vi "joystick control debugging.vi"() -> ()   [LabVIEW 2014]
uses:
  <vilib>/Utility/inputDevices.llb/joystickAcquire.vi
  <vilib>/Utility/inputDevices.llb/closeJoystick.vi
panel:
  out "device ID":refnum<k1>
  out "button info":T1
  out "device ID 2":refnum<k1>
  out "Value":T2(ring)
  out "JoystOffset":T3={"XOffset"=-99999, "YOffset"=-99999, "ZOffset"=-99999}
  out "RelJoyPos":T4
  in  "XMotorRef":refnum<k7>(container)
  in  "YMotorRef":refnum<k7>(container)
  in  "ZMotorRef":refnum<k7>(container)
  out "joystick info":T5(array[cluster])
  out "InstrumentMode":T2(ring)=enum."Shutdown"
  in  "InterfaceSelector":T6(tab)
  in  "GoToTopDisp":bool
  in  "GoToBottDisp":bool
  in  "GoToExpLoc":bool
  in  "SaveTopDisp":bool
  in  "SaveBottDisp":bool
  in  "SaveExpLoc":bool
  out "Top Dispenser":T7={"X Pos (mm)"=0.5532008, "Y Pos (mm)"=0.030929338, "Z Pos (mm)"=0.77973413} {"Y Pos (mm)" format="%.3f"; "Z Pos (mm)" format="%.3f"; "X Pos (mm)" format="%.3f"}
  out "Bottom Dispenser":T7={"X Pos (mm)"=0.600309, "Y Pos (mm)"=-1.1540928, "Z Pos (mm)"=0.7938141} {"Y Pos (mm)" format="%.3f"; "Z Pos (mm)" format="%.3f"; "X Pos (mm)" format="%.3f"}
  out "Experiment Region":T7={"X Pos (mm)"=1.4278219, "Y Pos (mm)"=-0.74810517, "Z Pos (mm)"=0.7938141} {"Y Pos (mm)" format="%.3f"; "Z Pos (mm)" format="%.3f"; "X Pos (mm)" format="%.3f"}
  in  "PreviewPanel":T8(tab)
  in  "Z Motor Settings":T9={"Joyst Min Signal"=10.0, "Joyst Max Signal"=30000.0, "Vmax (mm/s)"=0.005, "Acc (mm/s/s)"=0.2, "+ JoystDirection"=2, "- JoystDirection"=1} {"Acc (mm/s/s)" format="%#.3f"; "Vmax (mm/s)" format="%#.3f"}
  in  "Y Motor Settings":T9={"Joyst Min Signal"=10.0, "Joyst Max Signal"=20000.0, "Vmax (mm/s)"=0.03, "Acc (mm/s/s)"=0.5, "+ JoystDirection"=1, "- JoystDirection"=2} {"Acc (mm/s/s)" format="%#.3f"; "Vmax (mm/s)" format="%#.3f"}
  in  "X Motor Settings":T9={"Joyst Min Signal"=10.0, "Joyst Max Signal"=20000.0, "Vmax (mm/s)"=0.03, "Acc (mm/s/s)"=0.5, "+ JoystDirection"=2, "- JoystDirection"=1} {"Acc (mm/s/s)" format="%#.3f"; "Vmax (mm/s)" format="%#.3f"}
  in  "Motor Cruise Param":T10={"X Acc (mm/s^2)"=0.3, "X Vmax (mm/s)"=0.3, "Y Acc (mm/s^2)"=0.3, "Y Vmax (mm/s)"=0.3, "Z Acc (mm/s^2)"=0.1, "Z Vmax (mm/s)"=0.1}
  in  "Motor Limits":T11={"XMin"=-0.8, "XMax"=3.0, "YMin"=-2.0, "YMax"=2.0, "ZMin"=0.0, "ZMax"=2.0}
  in  "Steerable Mirror Calibration":T12={"Hor. Scaling (nm/V)"=760.0, "Vert. Scaling (nm/V)"=760.0, "Hor. Mirr. Offset (V)"=0.0, "Vert. Mirr. Offset (V)"=0.0}
  in  "Steerable \nTrap\n(F12)":bool
  in  "Fixed\nTrap\n(F11)":bool
  in  "Align Traps Vertically":bool
  in  "MaxHorizontalTrapSeparation":bool
  out "X Motor State":T13={"Direction"=0, "Vel (mm/s)"=0.0, "IsActive?"=FALSE, "Pos (mm)"=-0.2957381} {"Pos (mm)" format="%#.3f"; "Vel (mm/s)" format="%#.4f"}
  out "Y Motor State":T13={"Direction"=0, "Vel (mm/s)"=0.0, "IsActive?"=FALSE, "Pos (mm)"=0.016441232} {"Pos (mm)" format="%#.3f"; "Vel (mm/s)" format="%#.4f"}
  out "Z Motor State":T13={"Direction"=0, "Vel (mm/s)"=0.0, "IsActive?"=FALSE, "Pos (mm)"=-0.26253498} {"Pos (mm)" format="%#.3f"; "Vel (mm/s)" format="%#.4f"}
  out "Move Z":bool
  out "Move XY":bool
  in  "MotorLoopDelay":u32=100
  in  "PMVertSlider(V)":dbl(slide)=0.005145263671875 scale=0.0..10.0 scale format="%#_3f"
  in  "PMHorizSlider(V)":dbl(slide)=0.0045623779296875 scale=2.0..10.0
  out "Force TrapA":cluster{"x":dbl[], "y":dbl[]}[](graph)
  out "Noise-Ext":cluster{"x":dbl[], "y":dbl[]}[](graph)
  out "Force TrapB":cluster{"x":dbl[], "y":dbl[]}[](graph)
  out "IsOffsetModeActive?":bool caption="stop"
  # "Chamber Locations"
  # "Need a Button Here that would read the \nNormalized Offset and save it"
  # "Off"
  # "On"
  # "Off"
  # "On"
  # "Thorlabs Motor Status"
  # "Passive Mode"
  # "when I switch tabs from the passive mode to basic mode, the recording doesn't stop"
  # "The sliders don't do anything in passive mode, fix it"
  # "Whenever I click on Ackquire Offset, it goes back to the basic operation, then I have to ckick again"
  # "Trap Motion Control"
  # "Steerable Mirror Info"
  # "Zero-Force Offset Mode"
  # "High Frequency Data Acquisition"
  # "Adjust the length of acquisition time"
  # "Force-Extension Mode"
  # "Y"
  # "+"
  # "X"
  # "-"
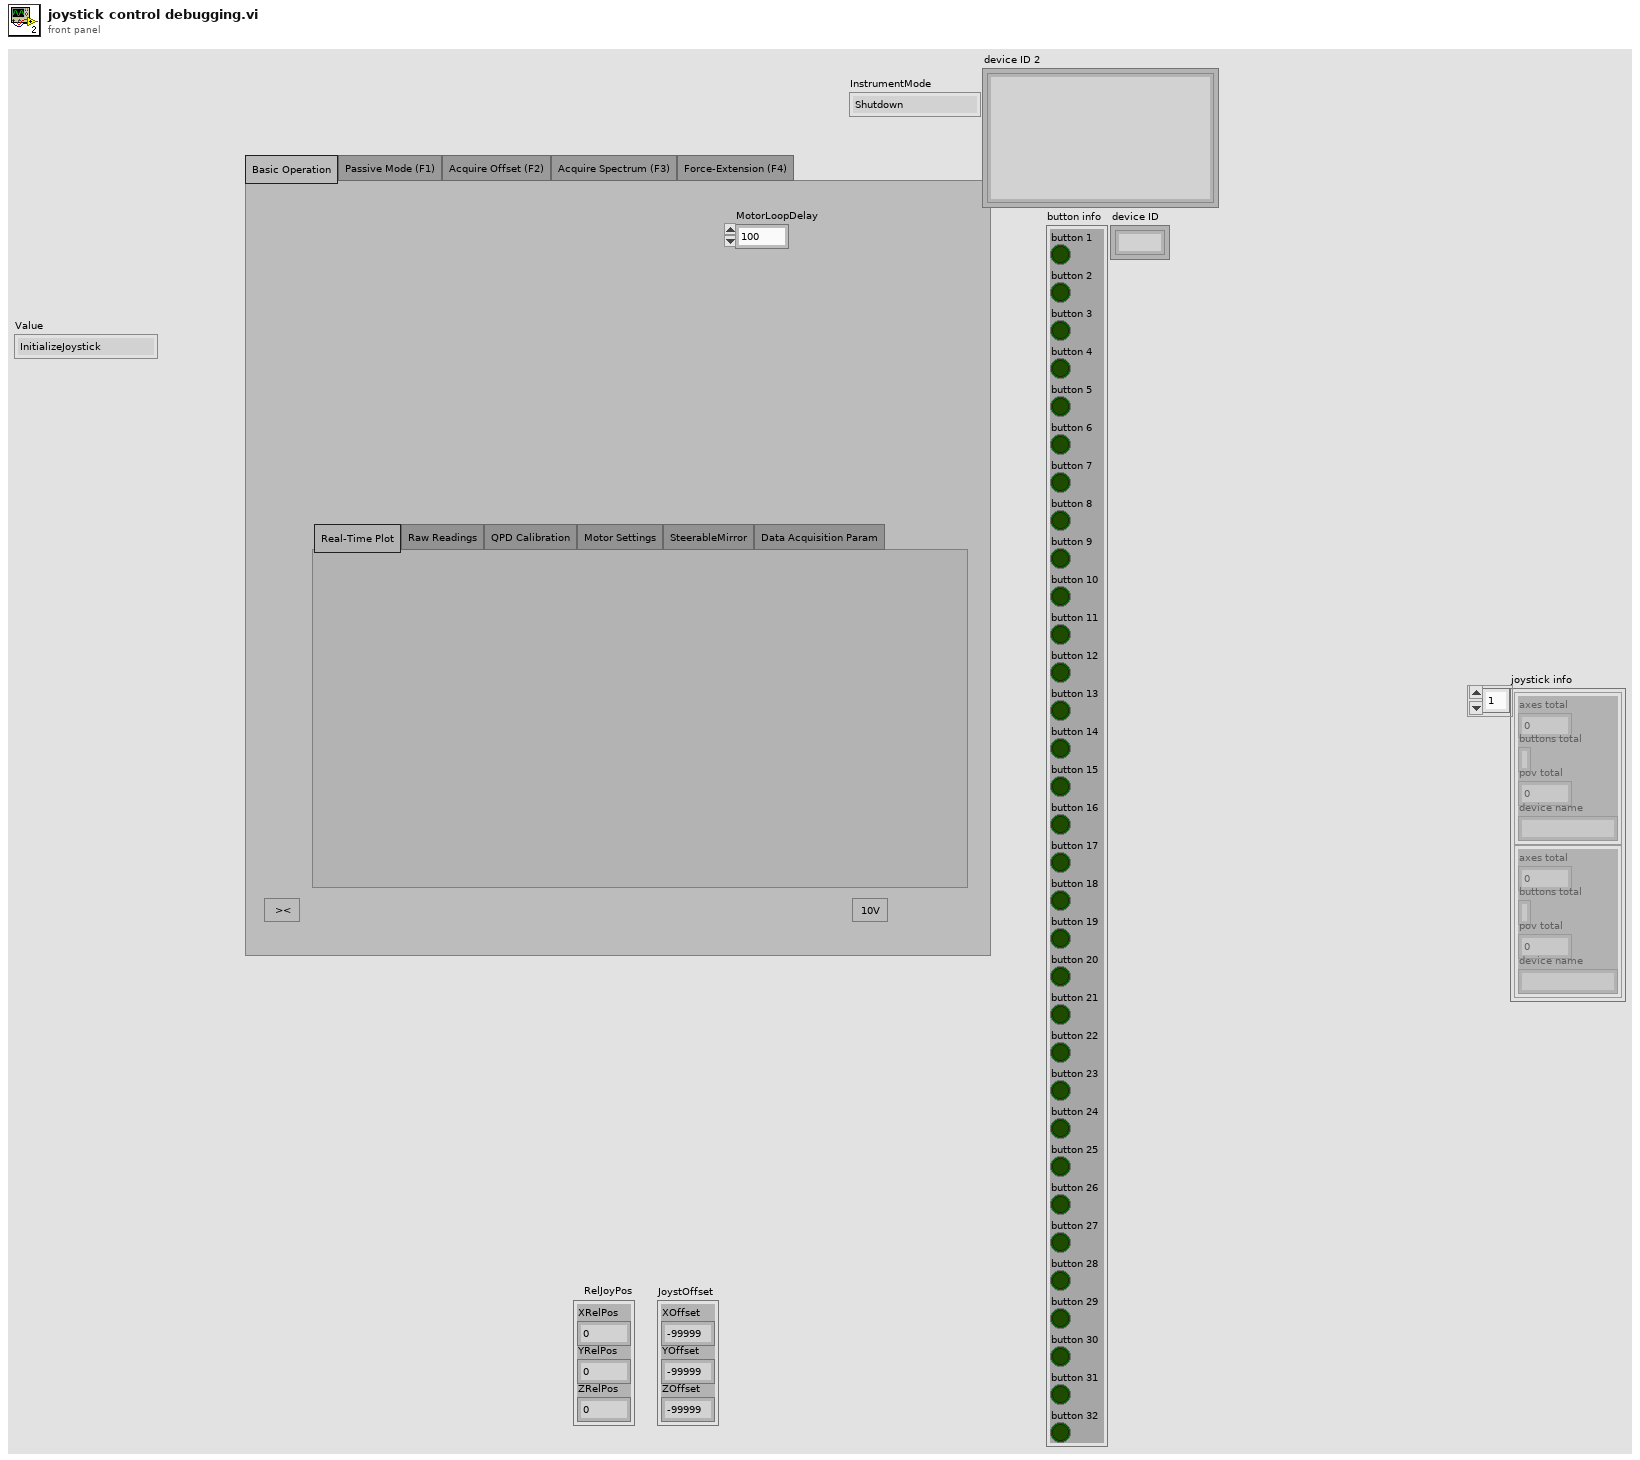
[diagram p1: front panel]
types:
  T1 = cluster{"button 1":bool, "button 2":bool, "button 3":bool, "button 4":bool, "button 5":bool, "button 6":bool, "button 7":bool, "button 8":bool, "button 9":bool, "button 10":bool, "button 11":bool, "button 12":bool, "button 13":bool, "button 14":bool, "button 15":bool, "button 16":bool, "button 17":bool, "button 18":bool, "button 19":bool, "button 20":bool, "button 21":bool, "button 22":bool, "button 23":bool, "button 24":bool, "button 25":bool, "button 26":bool, "button 27":bool, "button 28":bool, "button 29":bool, "button 30":bool, "button 31":bool, "button 32":bool}
  T2 = enum16{"InitializeJoystick", "InitializeMotors", "BasicMode", "PassiveMode", "AcquireOffsetMode", "AcquireSpectrumMode", "Force-ExtensionMode", "Shutdown"}
  T3 = cluster{"XOffset":i32, "YOffset":i32, "ZOffset":i32}
  T4 = cluster{"XRelPos":i32, "YRelPos":i32, "ZRelPos":i32}
  T5 = cluster{"axes total":u32, "buttons total":u32, "pov total":u32, "device name":string}[]
  T6 = enum32{"Basic Operation", "Passive Mode (F1)", "Acquire Offset (F2)", "Acquire Spectrum (F3)", "Force-Extension (F4)"}
  T7 = cluster{"X Pos (mm)":sgl, "Y Pos (mm)":sgl, "Z Pos (mm)":sgl}
  T8 = enum32{"Real-Time Plot", "Raw Readings", "QPD Calibration", "Motor Settings", "SteerableMirror", "Data Acquisition Param"}
  T9 = cluster{"Joyst Min Signal":dbl, "Joyst Max Signal":dbl, "Vmax (mm/s)":sgl, "Acc (mm/s/s)":sgl, "+ JoystDirection":i32, "- JoystDirection":i32}
  T10 = cluster{"X Acc (mm/s^2)":sgl, "X Vmax (mm/s)":sgl, "Y Acc (mm/s^2)":sgl, "Y Vmax (mm/s)":sgl, "Z Acc (mm/s^2)":sgl, "Z Vmax (mm/s)":sgl}
  T11 = cluster{"XMin":sgl, "XMax":sgl, "YMin":sgl, "YMax":sgl, "ZMin":sgl, "ZMax":sgl}
  T12 = cluster{"Hor. Scaling (nm/V)":dbl, "Vert. Scaling (nm/V)":dbl, "Hor. Mirr. Offset (V)":dbl, "Vert. Mirr. Offset (V)":dbl}
  T13 = cluster{"Direction":i32, "Vel (mm/s)":sgl, "IsActive?":bool, "Pos (mm)":sgl}
  T14 = cluster{"Motor Reference":refnum<k7>, "Motor Reference":refnum<k7>, "Motor Reference":refnum<k7>}
  T15 = cluster{"X axis":i32, "Y axis":i32, "Z axis":i32, "X axis rotation":i32, "Y axis rotation":i32, "Z axis rotation":i32, "U axis":i32, "V axis":i32}
  T16 = cluster{"XMotorRef":refnum<k7>, "YMotorRef":refnum<k7>, "ZMotorRef":refnum<k7>}
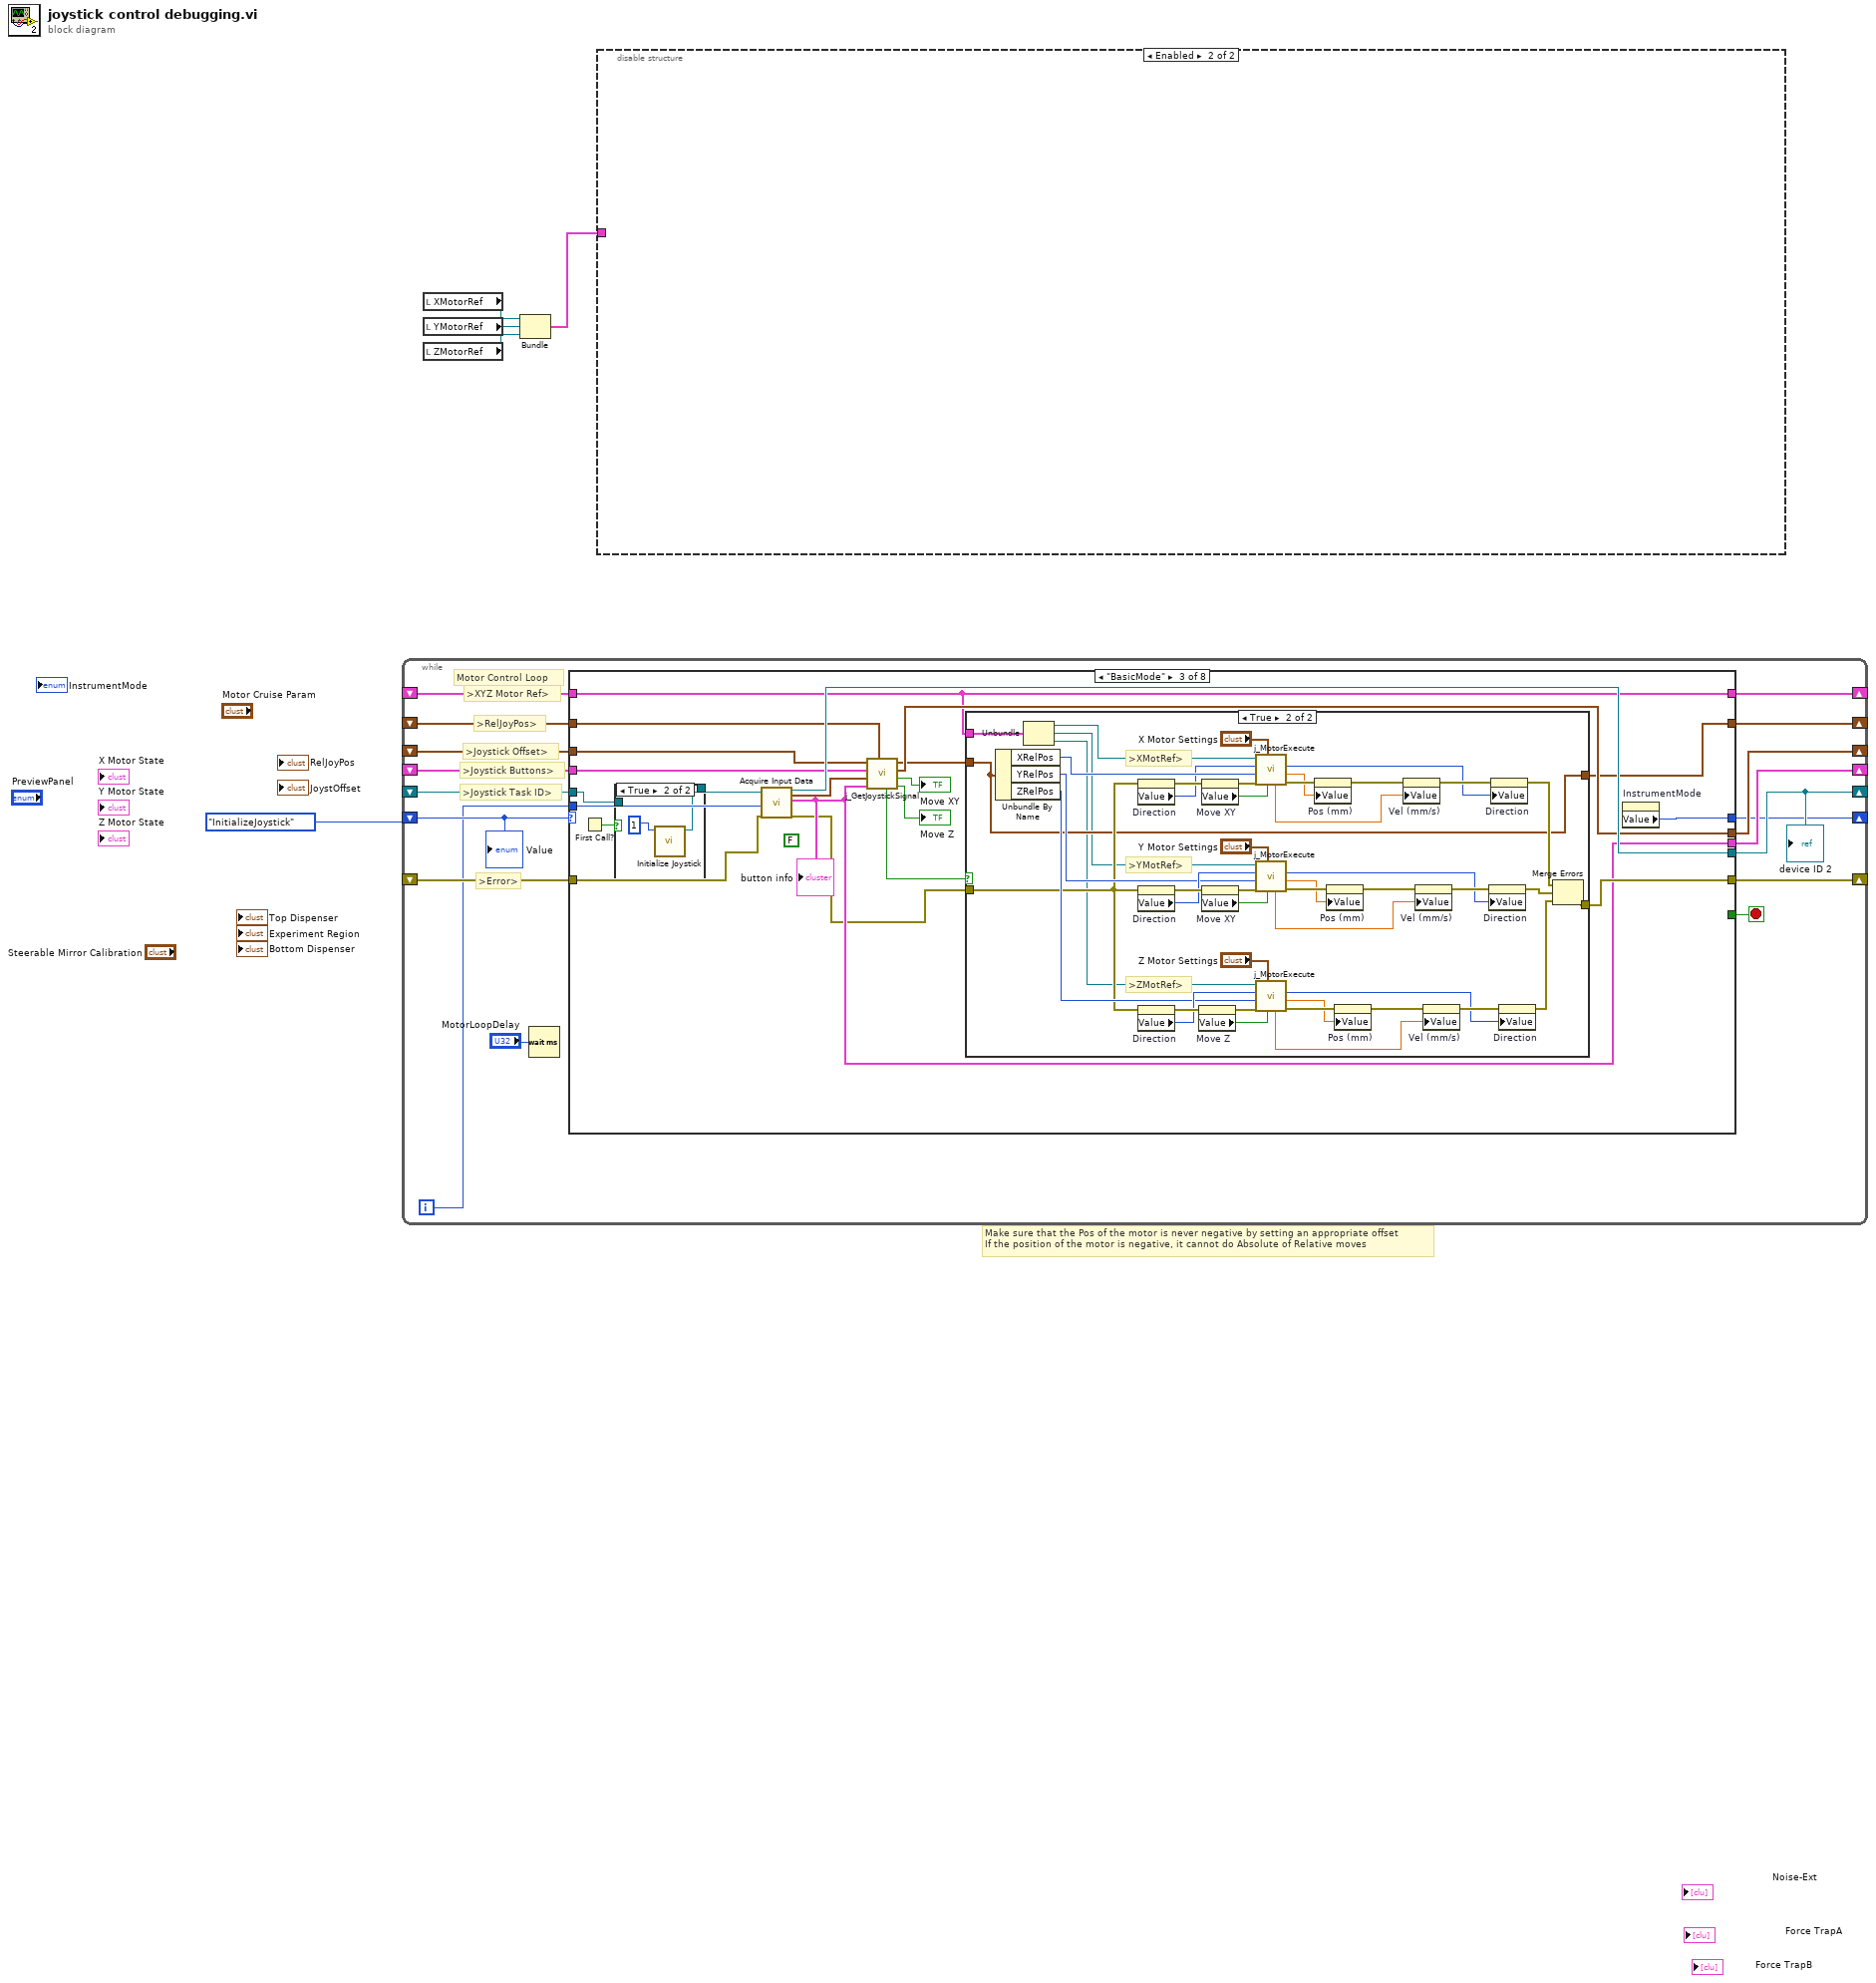
[diagram p0: block diagram]
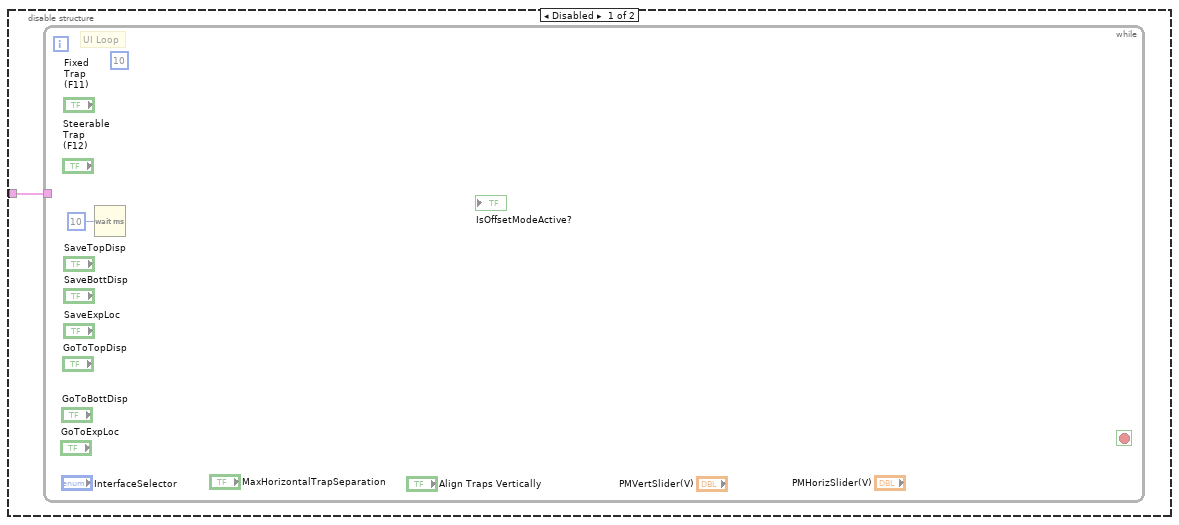
[diagram p2: hidden frame]
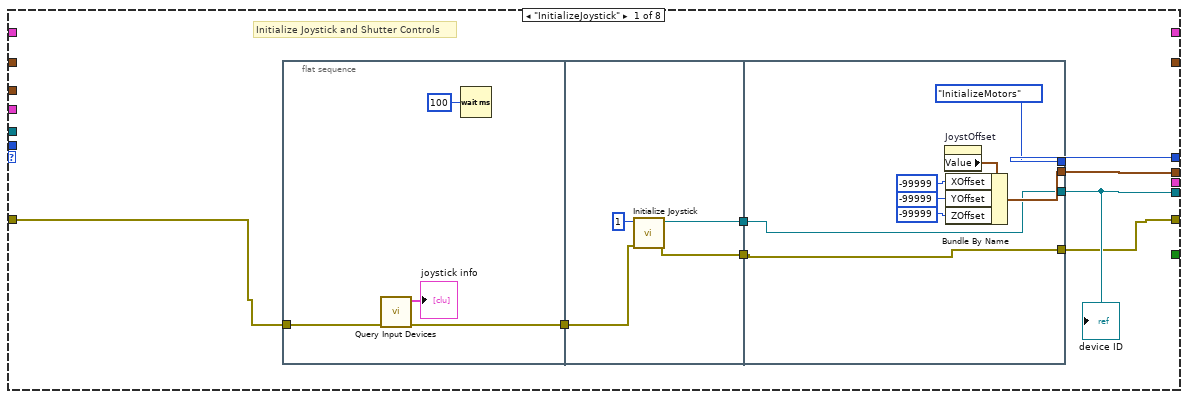
[diagram p3: hidden frame]
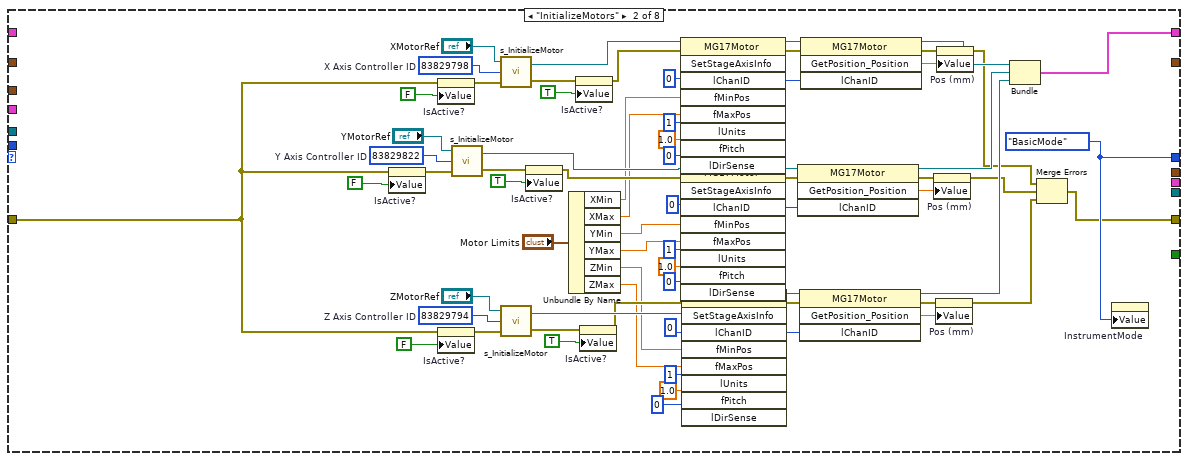
[diagram p4: hidden frame]
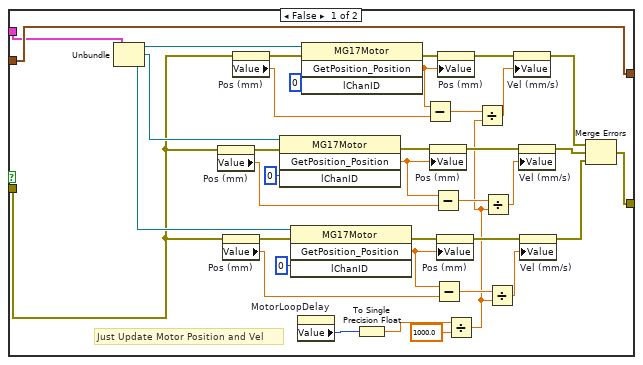
[diagram p6: hidden frame]
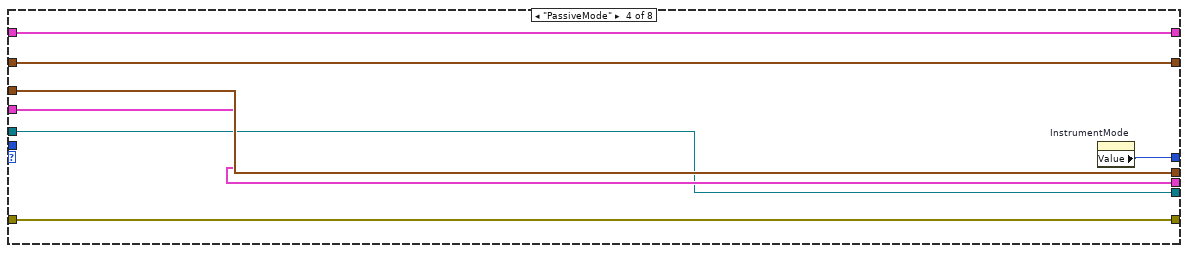
[diagram p7: hidden frame]
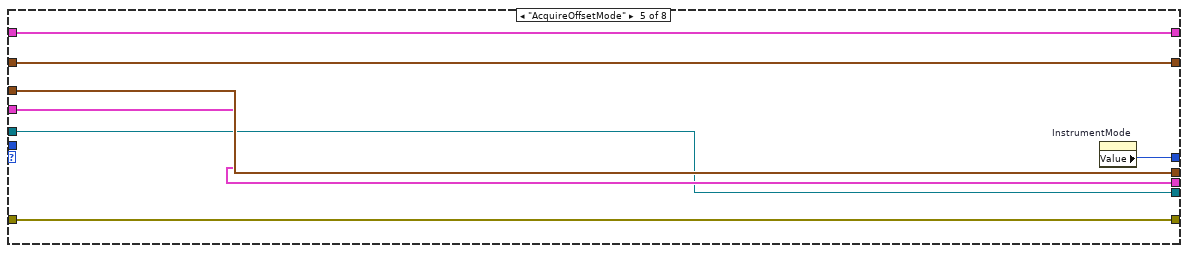
[diagram p8: hidden frame]
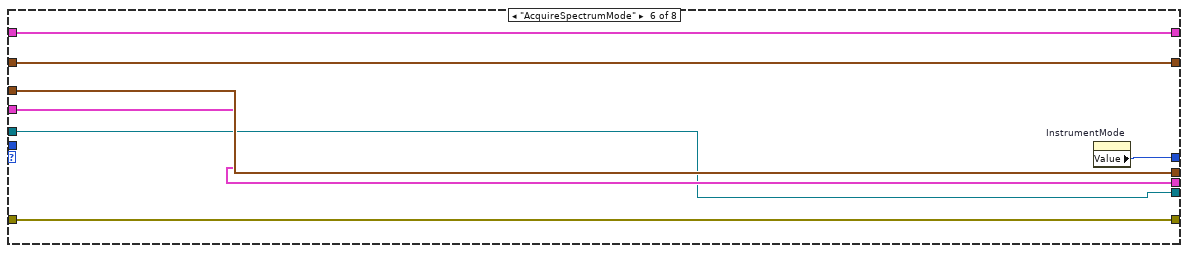
[diagram p9: hidden frame]
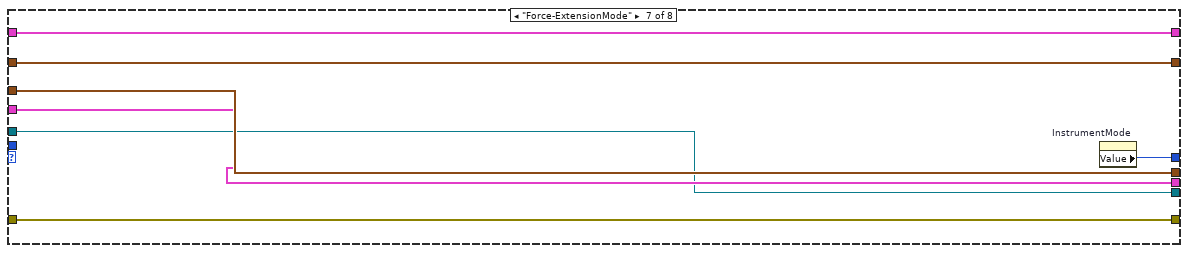
[diagram p10: hidden frame]
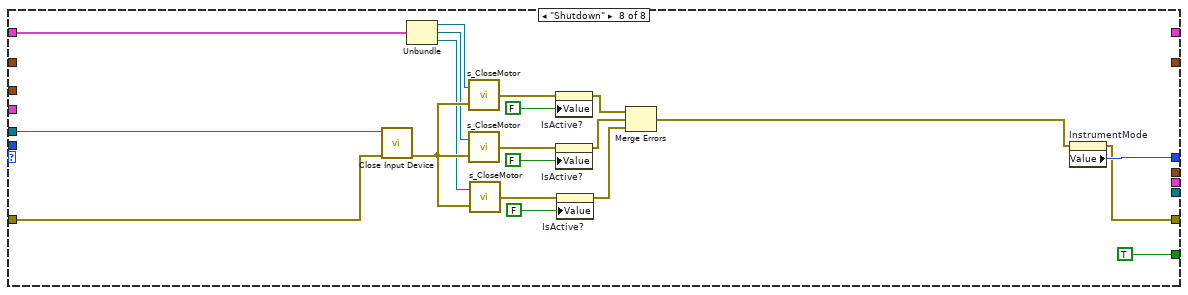
[diagram p11: hidden frame]
diagram:
  # "Make sure that the Pos of the motor is never negative by setting an appropriate offset\nIf the position of the motor is negative, it cannot do Absolute of Relative moves"
  n1 = while {
    shift-right: [w8] -> _
    shift-left: T2."InitializeJoystick" -> [w7]
    shift-right: [w22] -> _
    shift-left: _ -> [w15]
    shift-right: [w19] -> _
    shift-left: _ -> [w21]
    shift-right: [w20] -> _
    shift-left: _ -> [w18]
    shift-right: [w17] -> _
    shift-left: _ -> [w16]
    shift-right: [w14] -> _
    shift-left: _ -> [w11]
    shift-right: [w12] -> _
    shift-left: _ -> [w13]
    i -> [w6]
    stop <- w9 stop-if-true
    # "Motor Control Loop"
    # ">Joystick Offset>"
    # ">RelJoyPos>"
    # ">XYZ Motor Ref>"
    # ">Error>"
    # ">Joystick Task ID>"
    # ">Joystick Buttons>"
    n2 = Wait (ms)(milliseconds to wait="MotorLoopDelay") -> ()  [unwired: 1 out]
    n3 = case shown="\"BasicMode\"" w7 {
      tunnel: [w30 _ w133 w225 w232 w239 w246 _] -> w22
      tunnel: [w28 w48 w122 w229 w236 w243 w250 w269] -> w8
      tunnel: w21 -> [w27 w96 w135 w228 w235 w242 w249 w254]
      tunnel: [w29 _ w134 w223 w230 w237 w244 _] -> w20
      tunnel: [w26 w47 w126 w228 w235 w242 w249 w251] -> w19
      tunnel: w18 -> [_ _ w115 w223 w230 w237 w244 w253]
      tunnel: [_ _ w121 w224 w231 w238 w245 _] -> w17
      tunnel: w16 -> [_ _ w120 w224 w231 w238 w245 _]
      tunnel: w15 -> [_ _ w131 w225 w232 w239 w246 _]
      tunnel: [_ _ _ _ _ _ _ TRUE ("status")] -> w9
      tunnel: [_ w95 w125 w227 w234 w241 w248 _] -> w14
      tunnel: w11 -> [_ _ w125 w227 w234 w241 w248 w255]
      tunnel: [_ _ w123 w226 w233 w240 w247 _] -> w12
      tunnel: w13 -> [_ _ w132 w226 w233 w240 w247 _]
      tunnel: w6 -> [_ _ w118 _ _ _ _ _]
      frame "InitializeJoystick" {
        # "Initialize Joystick and Shutter Controls"
        n4 = flat-sequence {
          tunnel: w27 -> [w32]
          tunnel: [w31] -> w25
          tunnel: w25 -> [w37]
          tunnel: [w36] -> w24
          tunnel: [w35] -> w23
          tunnel: [w43] -> w30
          tunnel: [w39] -> w29
          tunnel: [T2."InitializeMotors"] -> w28
          tunnel: w24 -> [w40]
          tunnel: [w40] -> w26
          tunnel: w23 -> [w39]
          frame #0 {
            n5 = call <vilib>:"Query Input Devices.vi"("error in (no error)"=w32) -> ("error out"=w31:errorcluster, "joystick info"=→"joystick info":T5)  [unwired: 7 in, 2 out]
            n6 = Wait (ms)(milliseconds to wait=u32 100) -> ()  [unwired: 1 out]
          }
          frame #1 {
            n7 = call <vilib>:"Initialize Joystick.vi"("error in (no error)"=w37, "device index"=1) -> ("error out"=w36:errorcluster, "device ID"=w35:refnum<k1>)  [unwired: 8 in]
          }
          frame #2 {
            n8 = property on="JoystOffset" class="Clust (strict)"() -> ("Value"=w42:T3)  [unwired: 2 in, 2 out]
            n9 = Bundle By Name(cluster=w42, "XOffset"=-99999, "YOffset"=-99999, "ZOffset"=-99999) -> (w43:T3)
          }
        }
        "device ID" <- w29
      }
      frame "InitializeMotors" {
        w48 = T2."BasicMode"
        w100 = 83829794  # Z Axis Controller ID
        w106 = 83829822  # Y Axis Controller ID
        w112 = 83829798  # X Axis Controller ID
        n10 = property on="IsActive?" class="Bool (strict)"(error in=w96, "Value"=FALSE ("IsYMotorActive?")) -> (error out=w107:errorcluster)  [unwired: 1 in, 1 out]
        n11 = property on="IsActive?" class="Bool (strict)"(error in=w96, "Value"=FALSE ("IsYMotorActive?")) -> (error out=w113:errorcluster)  [unwired: 1 in, 1 out]
        n12 = property on="IsActive?" class="Bool (strict)"(error in=w96, "Value"=FALSE ("IsYMotorActive?")) -> (error out=w101:errorcluster)  [unwired: 1 in, 1 out]
        n13 = call "s_InitializeMotor.vi"("Error In"=w107, "Servo Controller  ID"=w106, "Motor Reference In"="YMotorRef") -> ("Error Out"=w108:errorcluster, "Motor Reference"=w90:refnum<k7>)
        n14 = call "s_InitializeMotor.vi"("Error In"=w113, "Servo Controller  ID"=w112, "Motor Reference In"="XMotorRef") -> ("Error Out"=w114:errorcluster, "Motor Reference"=w94:refnum<k7>)
        n15 = call "s_InitializeMotor.vi"("Error In"=w101, "Servo Controller  ID"=w100, "Motor Reference In"="ZMotorRef") -> ("Error Out"=w102:errorcluster, "Motor Reference"=w87:refnum<k7>)
        n16 = property on="IsActive?" class="Bool (strict)"(error in=w108, "Value"=TRUE ("IsYMotorActive?")) -> (error out=w89:errorcluster)  [unwired: 1 in, 1 out]
        n17 = Unbundle By Name("Motor Limits") -> ("XMin"=w54:sgl, "XMax"=w53:sgl, "YMin"=w52:sgl, "YMax"=w51:sgl, "ZMin"=w50:sgl, "ZMax"=w49:sgl)
        n18 = property on="IsActive?" class="Bool (strict)"(error in=w114, "Value"=TRUE ("IsYMotorActive?")) -> (error out=w92:errorcluster)  [unwired: 1 in, 1 out]
        n19 = property on="IsActive?" class="Bool (strict)"(error in=w102, "Value"=TRUE ("IsYMotorActive?")) -> (error out=w86:errorcluster)  [unwired: 1 in, 1 out]
        n20 = invoke class="MG17Motor" method="SetStageAxisInfo"(reference=w94, error in=w92, "lChanID"=0, "fMinPos"=w54, "fMaxPos"=w53, "lUnits"=1, "fPitch"=sgl 1.0, "lDirSense"=0) -> (reference out=w85:refnum<k7>, error out=w84:errorcluster, "lChanID"=w83:i32)  [unwired: 1 in, 6 out]
        n21 = invoke class="MG17Motor" method="SetStageAxisInfo"(reference=w90, error in=w89, "lChanID"=0, "fMinPos"=w52, "fMaxPos"=w51, "lUnits"=1, "fPitch"=sgl 1.0, "lDirSense"=0) -> (reference out=w77:refnum<k7>, error out=w76:errorcluster, "lChanID"=w75:i32)  [unwired: 1 in, 6 out]
        n22 = invoke class="MG17Motor" method="SetStageAxisInfo"(reference=w87, error in=w86, "lChanID"=0, "fMinPos"=w50, "fMaxPos"=w49, "lUnits"=1, "fPitch"=sgl 1.0, "lDirSense"=0) -> (reference out=w72:refnum<k7>, error out=w71:errorcluster, "lChanID"=w70:i32)  [unwired: 1 in, 6 out]
        n23 = invoke class="MG17Motor" method="GetPosition_Position"(reference=w77, error in=w76, "lChanID"=w75) -> (reference out=w69:refnum<k7>, error out=w79:errorcluster, "GetPosition_Position"=w78:sgl)  [unwired: 1 in, 1 out]
        n24 = invoke class="MG17Motor" method="GetPosition_Position"(reference=w72, error in=w71, "lChanID"=w70) -> (reference out=w68:refnum<k7>, error out=w74:errorcluster, "GetPosition_Position"=w73:sgl)  [unwired: 1 in, 1 out]
        n25 = invoke class="MG17Motor" method="GetPosition_Position"(reference=w85, error in=w84, "lChanID"=w83) -> (reference out=w82:refnum<k7>, error out=w81:errorcluster, "GetPosition_Position"=w80:sgl)  [unwired: 1 in, 1 out]
        n26 = property on="Pos (mm)" class="DigNum (strict)"(error in=w79, "Value"=w78) -> (error out=w67:errorcluster)  [unwired: 1 in, 1 out]
        n27 = property on="Pos (mm)" class="DigNum (strict)"(error in=w74, "Value"=w73) -> (error out=w65:errorcluster)  [unwired: 1 in, 1 out]
        n28 = property on="Pos (mm)" class="DigNum (strict)"(error in=w81, "Value"=w80) -> (error out=w66:errorcluster)  [unwired: 1 in, 1 out]
        n29 = Bundle("Motor Reference"=w82, "Motor Reference"=w69, "Motor Reference"=w68) -> (w95:T14)  [unwired: 1 in]
        n30 = Merge Errors(w66, w67, w65) -> (w47:errorcluster)
        n31 = property on="InstrumentMode" class="Enum (strict)"("Value"=w48) -> ()  [unwired: 2 in, 2 out]
      }
      frame "BasicMode" {
        (unwired) FALSE
        n32 = First Call?() -> (First Call?: T/F=w116:bool)
        n33 = case shown="True" w116 {
          tunnel: [w136 w137] -> w117
          tunnel: w115 -> [w136 _]
          frame False {
          }
          frame True {
            n34 = call <vilib>:"Initialize Joystick.vi"("device index"=1) -> ("device ID"=w137:refnum<k1>)  [unwired: 9 in, 1 out]
          }
        }
        n35 = call-poly <vilib>:"Acquire Input Data.vi"("device ID"=w117, "Numeric"=w118, "error in (no error)"=w135) -> ("device ID 2"=w134:refnum<k1>, "axis info"=w130:T15, "button info"=w121:T1, "error out"=w119:errorcluster)  [unwired: 12 in, 1 out]
        "button info" <- w121
        n36 = call "j_GetJoystickSignal.vi"("RelJoyPos In"=w132, "NewJoystButtInfo"=w121, "NewJoystAxisInfo"=w130, "OldJoystButtInfo"=w120, "OldJoystickOffset"=w131) -> ("MoveZ"=→"Move Z":bool, "MoveXY"=→"Move XY":bool, "Joystick Offset"=w133:T3, "RelJoyPos"=w127:T4, "TalkToMotors?"=w124:bool)
        n37 = case shown="True" w124 {
          tunnel: w127 -> [w176 w180]
          tunnel: [w165 w197] -> w126
          tunnel: w125 -> [w175 w183]
          tunnel: w119 -> [w149 w182]
          tunnel: [w176 w180] -> w123
          frame False {
            # "Just Update Motor Position and Vel"
            n38 = Unbundle(w175) -> ("Motor Reference"=w174:refnum<k7>, "Motor Reference"=w167:refnum<k7>, "Motor Reference"=w166:refnum<k7>)
            n39 = property on="Pos (mm)" class="DigNum (strict)"(error in=w149) -> (error out=w157:errorcluster, "Value"=w154:sgl)  [unwired: 1 in, 1 out]
            n40 = property on="Pos (mm)" class="DigNum (strict)"(error in=w149) -> (error out=w150:errorcluster, "Value"=w147:sgl)  [unwired: 1 in, 1 out]
            n41 = property on="Pos (mm)" class="DigNum (strict)"(error in=w149) -> (error out=w158:errorcluster, "Value"=w163:sgl)  [unwired: 1 in, 1 out]
            n42 = invoke class="MG17Motor" method="GetPosition_Position"(reference=w167, error in=w157, "lChanID"=0) -> (error out=w170:errorcluster, "GetPosition_Position"=w155:sgl)  [unwired: 1 in, 2 out]
            n43 = invoke class="MG17Motor" method="GetPosition_Position"(reference=w166, error in=w150, "lChanID"=0) -> (error out=w168:errorcluster, "GetPosition_Position"=w146:sgl)  [unwired: 1 in, 2 out]
            n44 = property on="MotorLoopDelay" class="DigNum (strict)"() -> ("Value"=w142:u32)  [unwired: 2 in, 2 out]
            n45 = invoke class="MG17Motor" method="GetPosition_Position"(reference=w174, error in=w158, "lChanID"=0) -> (error out=w172:errorcluster, "GetPosition_Position"=w164:sgl)  [unwired: 1 in, 2 out]
            n46 = To Single Precision Float(number=w142) -> (single precision float=w141:sgl)
            n47 = Subtract(x=w164, y=w163) -> (x-y=w162:sgl)
            n48 = property on="Pos (mm)" class="DigNum (strict)"(error in=w170, "Value"=w155) -> (error out=w153:errorcluster)  [unwired: 1 in, 1 out]
            n49 = Subtract(x=w155, y=w154) -> (x-y=w156:sgl)
            n50 = Subtract(x=w146, y=w147) -> (x-y=w148:sgl)
            n51 = property on="Pos (mm)" class="DigNum (strict)"(error in=w168, "Value"=w146) -> (error out=w145:errorcluster)  [unwired: 1 in, 1 out]
            n52 = property on="Pos (mm)" class="DigNum (strict)"(error in=w172, "Value"=w164) -> (error out=w160:errorcluster)  [unwired: 1 in, 1 out]
            n53 = Divide(x=w141, y=sgl 1000.0) -> (x/y=w139:sgl)
            n54 = Divide(x=w162, y=w139) -> (x/y=w161:sgl)
            n55 = Divide(x=w156, y=w139) -> (x/y=w152:sgl)
            n56 = Divide(x=w148, y=w139) -> (x/y=w144:sgl)
            n57 = property on="Vel (mm/s)" class="DigNum (strict)"(error in=w160, "Value"=w161) -> (error out=w159:errorcluster)  [unwired: 1 in, 1 out]
            n58 = property on="Vel (mm/s)" class="DigNum (strict)"(error in=w153, "Value"=w152) -> (error out=w151:errorcluster)  [unwired: 1 in, 1 out]
            n59 = property on="Vel (mm/s)" class="DigNum (strict)"(error in=w145, "Value"=w144) -> (error out=w143:errorcluster)  [unwired: 1 in, 1 out]
            n60 = Merge Errors(w159, w151, w143) -> (w165:errorcluster)
          }
          frame True {
            # ">ZMotRef>"
            # ">YMotRef>"
            # ">XMotRef>"
            n61 = Unbundle By Name(w180) -> ("XRelPos"=w213:i32, "YRelPos"=w199:i32, "ZRelPos"=w184:i32)
            n62 = Unbundle(w183) -> ("Motor Reference"=w179:refnum<k7>, "Motor Reference"=w178:refnum<k7>, "Motor Reference"=w177:refnum<k7>)
            n63 = property on="Direction" class="DigNum (strict)"(error in=w182) -> (error out=w212:errorcluster, "Value"=w211:i32)  [unwired: 1 in, 1 out]
            n64 = property on="Direction" class="DigNum (strict)"(error in=w182) -> (error out=w202:errorcluster, "Value"=w201:i32)  [unwired: 1 in, 1 out]
            n65 = property on="Direction" class="DigNum (strict)"(error in=w182) -> (error out=w187:errorcluster, "Value"=w186:i32)  [unwired: 1 in, 1 out]
            n66 = property on="Move Z" class="Bool (strict)"(error in=w187) -> (error out=w195:errorcluster, "Value"=w194:bool)  [unwired: 1 in, 1 out]
            n67 = property on="Move XY" class="Bool (strict)"(error in=w212) -> (error out=w221:errorcluster, "Value"=w220:bool)  [unwired: 1 in, 1 out]
            n68 = property on="Move XY" class="Bool (strict)"(error in=w202) -> (error out=w210:errorcluster, "Value"=w209:bool)  [unwired: 1 in, 1 out]
            n69 = call "j_MotorExecute.vi"("MoveChamber?"=w220, "Axis Motor Settings"="X Motor Settings", "Error In"=w221, "JoystRelPos"=w213, "Motor's Old Direction"=w211, "Motor Reference In"=w179) -> ("Error Out"=w216:errorcluster, "Motor Position (mm)"=w215:sgl, "Motor's New Direction"=w214:i32, "Motor Velocity (mm/s)"=w217:sgl)  [unwired: 1 out]
            n70 = call "j_MotorExecute.vi"("MoveChamber?"=w209, "Axis Motor Settings"="Y Motor Settings", "Error In"=w210, "JoystRelPos"=w199, "Motor's Old Direction"=w201, "Motor Reference In"=w178) -> ("Error Out"=w205:errorcluster, "Motor Position (mm)"=w204:sgl, "Motor's New Direction"=w203:i32, "Motor Velocity (mm/s)"=w206:sgl)  [unwired: 1 out]
            n71 = call "j_MotorExecute.vi"("MoveChamber?"=w194, "Axis Motor Settings"="Z Motor Settings", "Error In"=w195, "JoystRelPos"=w184, "Motor's Old Direction"=w186, "Motor Reference In"=w177) -> ("Error Out"=w190:errorcluster, "Motor Position (mm)"=w189:sgl, "Motor's New Direction"=w188:i32, "Motor Velocity (mm/s)"=w191:sgl)  [unwired: 1 out]
            n72 = property on="Pos (mm)" class="DigNum (strict)"(error in=w216, "Value"=w215) -> (error out=w218:errorcluster)  [unwired: 1 in, 1 out]
            n73 = property on="Pos (mm)" class="DigNum (strict)"(error in=w205, "Value"=w204) -> (error out=w207:errorcluster)  [unwired: 1 in, 1 out]
            n74 = property on="Pos (mm)" class="DigNum (strict)"(error in=w190, "Value"=w189) -> (error out=w192:errorcluster)  [unwired: 1 in, 1 out]
            n75 = property on="Vel (mm/s)" class="DigNum (strict)"(error in=w218, "Value"=w217) -> (error out=w219:errorcluster)  [unwired: 1 in, 1 out]
            n76 = property on="Vel (mm/s)" class="DigNum (strict)"(error in=w207, "Value"=w206) -> (error out=w208:errorcluster)  [unwired: 1 in, 1 out]
            n77 = property on="Vel (mm/s)" class="DigNum (strict)"(error in=w192, "Value"=w191) -> (error out=w193:errorcluster)  [unwired: 1 in, 1 out]
            n78 = property on="Direction" class="DigNum (strict)"(error in=w208, "Value"=w203) -> (error out=w196:errorcluster)  [unwired: 1 in, 1 out]
            n79 = property on="Direction" class="DigNum (strict)"(error in=w219, "Value"=w214) -> (error out=w198:errorcluster)  [unwired: 1 in, 1 out]
            n80 = property on="Direction" class="DigNum (strict)"(error in=w193, "Value"=w188) -> (error out=w181:errorcluster)  [unwired: 1 in, 1 out]
            n81 = Merge Errors(w198, w196, w181) -> (w197:errorcluster)
          }
        }
        n82 = property on="InstrumentMode" class="Enum (strict)"() -> ("Value"=w122:T2)  [unwired: 2 in, 2 out]
      }
      frame "PassiveMode" {
        n83 = property on="InstrumentMode" class="Enum (strict)"() -> ("Value"=w229:T2)  [unwired: 2 in, 2 out]
      }
      frame "AcquireOffsetMode" {
        n84 = property on="InstrumentMode" class="Enum (strict)"() -> ("Value"=w236:T2)  [unwired: 2 in, 2 out]
      }
      frame "AcquireSpectrumMode" {
        n85 = property on="InstrumentMode" class="Enum (strict)"() -> ("Value"=w243:T2)  [unwired: 2 in, 2 out]
      }
      frame "Force-ExtensionMode" {
        n86 = property on="InstrumentMode" class="Enum (strict)"() -> ("Value"=w250:T2)  [unwired: 2 in, 2 out]
      }
      frame "Shutdown" {
        n87 = call-poly <vilib>:"Close Input Device.vi"("error in (no error)"=w254, "device ID"=w253) -> ("error out"=w262:errorcluster)  [unwired: 8 in]
        n88 = Unbundle(w255) -> ("Motor Reference"=w258:refnum<k7>, "Motor Reference"=w257:refnum<k7>, "Motor Reference"=w256:refnum<k7>)
        n89 = call "s_CloseMotor.vi"("Error In"=w262, "Motor Reference In"=w258) -> ("Error Out"=w267:errorcluster)
        n90 = call "s_CloseMotor.vi"("Error In"=w262, "Motor Reference In"=w257) -> ("Error Out"=w265:errorcluster)
        n91 = call "s_CloseMotor.vi"("Error In"=w262, "Motor Reference In"=w256) -> ("Error Out"=w263:errorcluster)
        n92 = property on="IsActive?" class="Bool (strict)"(error in=w267, "Value"=FALSE ("IsYMotorActive?")) -> (error out=w261:errorcluster)  [unwired: 1 in, 1 out]
        n93 = property on="IsActive?" class="Bool (strict)"(error in=w265, "Value"=FALSE ("IsYMotorActive?")) -> (error out=w260:errorcluster)  [unwired: 1 in, 1 out]
        n94 = property on="IsActive?" class="Bool (strict)"(error in=w263, "Value"=FALSE ("IsYMotorActive?")) -> (error out=w259:errorcluster)  [unwired: 1 in, 1 out]
        n95 = Merge Errors(w261, w260, w259) -> (w252:errorcluster)
        n96 = property on="InstrumentMode" class="Enum (strict)"(error in=w252) -> (error out=w251:errorcluster, "Value"=w269:T2)  [unwired: 1 in, 1 out]
      }
    }
    "device ID 2" <- w20
    "Value" <- w7
  }
  n97 = local read "XMotorRef"() -> (w5:refnum<k7>)
  n98 = local read "YMotorRef"() -> (w4:refnum<k7>)
  n99 = local read "ZMotorRef"() -> (w3:refnum<k7>)
  n100 = Bundle("XMotorRef"=w5, "YMotorRef"=w4, "ZMotorRef"=w3) -> (w2:T16)  [unwired: 1 in]
  n101 = disable-structure shown="Enabled" {
    disable-tunnel: w2 -> [w271 _]
    frame Disabled {
      n102 = while {
        tunnel: w271 -> [_]
        stop <- _ stop-if-true
        (unwired) 10
        # "UI Loop"
        n103 = Wait (ms)(milliseconds to wait=u32 10) -> ()  [unwired: 1 out]
      }
    }
    frame Enabled {
    }
  }
